vi "_Validate Parameter.vi"(6 "Parameter":T1 {"Expt"."Mass Range"."Resolution Type" items=["High/High", "Medium/Medium", "Low/Low", "High/Medium", "High/Low", "Medium/High", "Medium/Low", "Low/High", "Low/Medium"]}, 9 "error in (no error)":errorcluster) -> (0 "Ch ID":i32[](array[numeric]), 1 "General Param":i32[](array[numeric]), 2 "RunMode":i32, 3 "error out":errorcluster, 4 "Low Values":i32[](array[numeric]), 5 "High Values (DAC)":i32[](array[numeric]))   [LabVIEW 2012]
uses:
  Type/_RT Parameter.ctl
  Type/_RT Active Ch.ctl
  Type/_RT Expt.ctl
  Type/_Run Mode.ctl
  Type/_RT Mass Range.ctl
  Type/_RT Res Type.ctl
  _RT Global.vi
panel:
  # "General Parameters:\n===============\nRun Mode\n# of Ch's\nHigh Level Time (uS) / Q1 Pol\nLow Level Time (uS) / Q2 Pol"
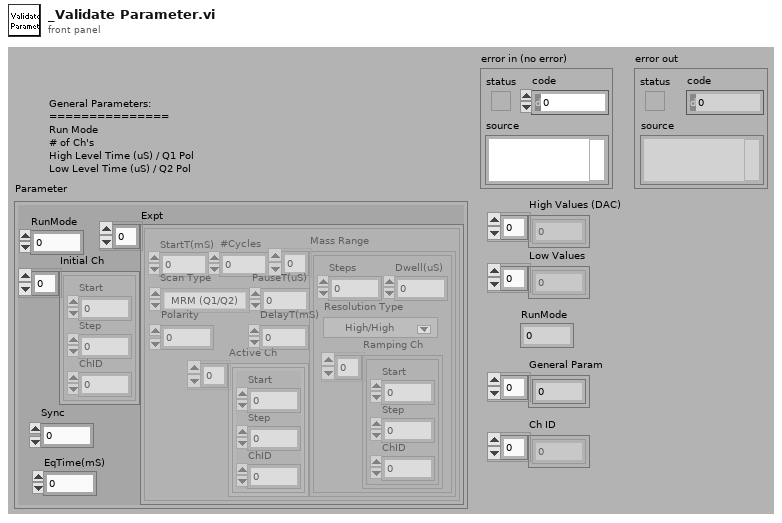
[diagram p1: front panel]
types:
  T1 = typedef "_RT Parameter.ctl" = cluster{"RunMode":i32, "Initial Ch":T2[], "Sync":u8, "Expt":T3[], "EqTime(mS)":i32}
  T2 = typedef "_RT Active Ch.ctl" = cluster{"Start":i32, "Step":i32, "ChID":i32}
  T3 = typedef "_RT Expt.ctl" = cluster{"StartT(mS)":i32, "#Cycles":i32, "Scan Type":T4, "PauseT(uS)":i32, "Polarity":u8, "DelayT(mS)":i32, "Active Ch":T2[], "Mass Range":T5[]}
  T4 = typedef "_Run Mode.ctl" = enum16{"MRM (Q1/Q2)", "Q1 Scan", "Q1 SRM", "Q2 Scan", "Q2 SRM", "Product Scan", "Precursor Scan", "Neutral Loss", "Neutral Gain"}
  T5 = typedef "_RT Mass Range.ctl" = cluster{"Steps":i32, "Dwell(uS)":i32, "Resolution Type":T6, "Ramping Ch":T2[]}
  T6 = typedef "_RT Res Type.ctl" = u16
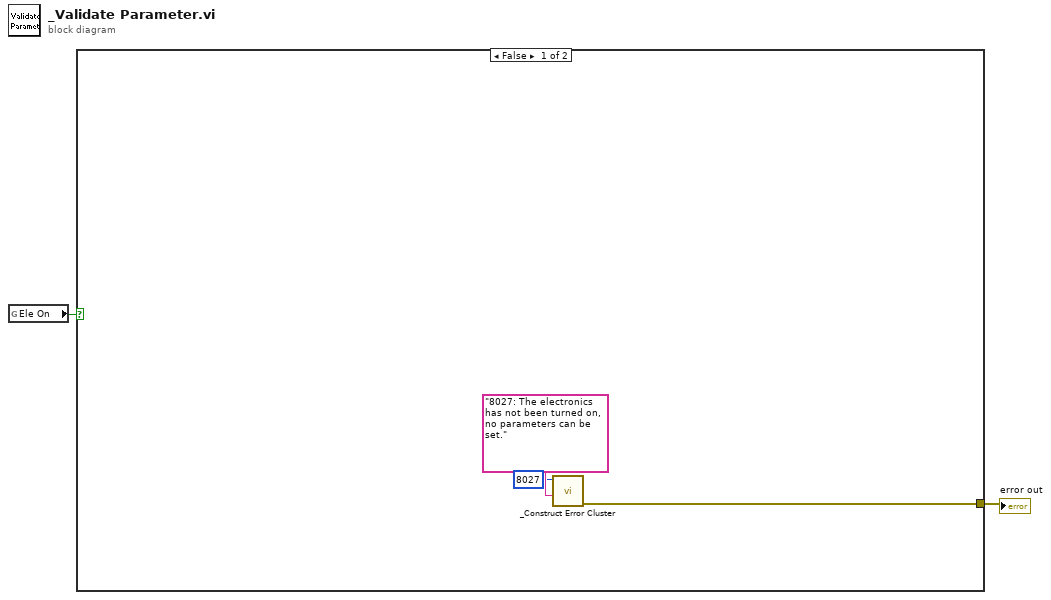
[diagram p0: block diagram]
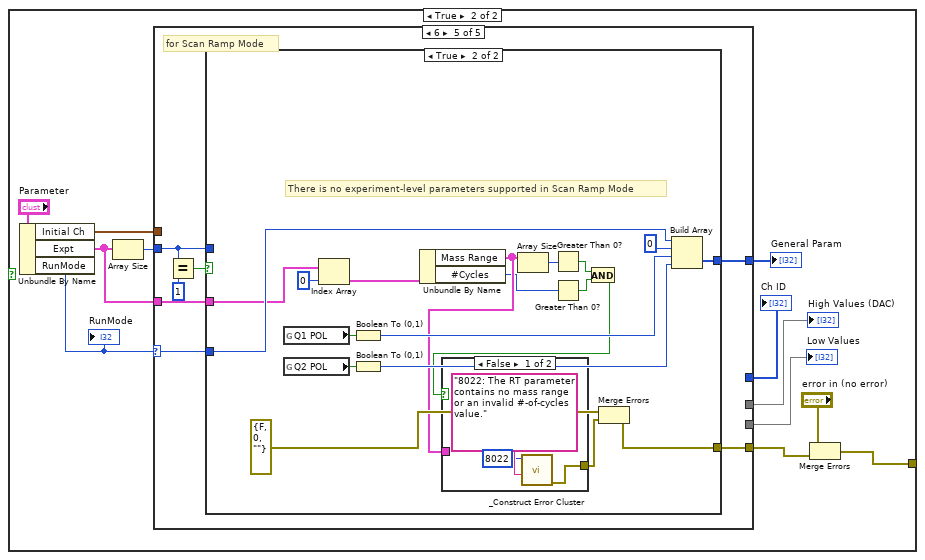
[diagram p2: hidden frame]
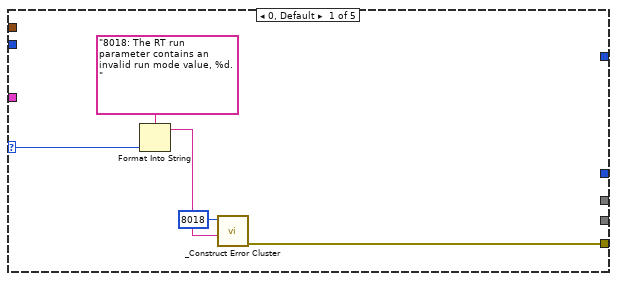
[diagram p3: hidden frame]
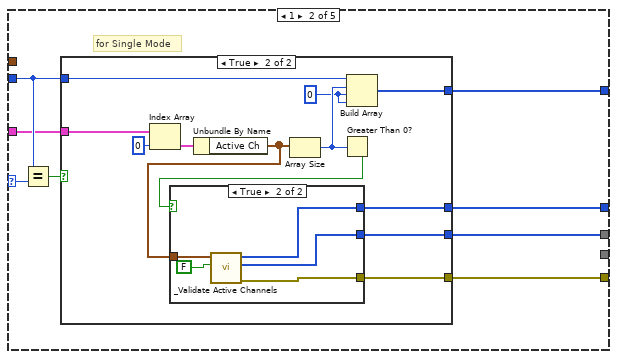
[diagram p4: hidden frame]
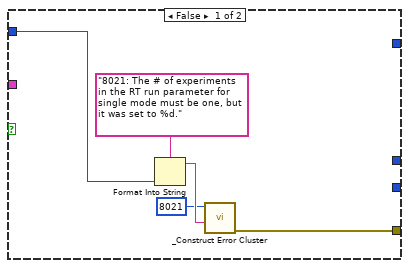
[diagram p5: hidden frame]
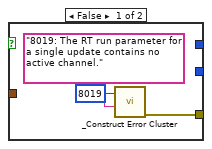
[diagram p6: hidden frame]
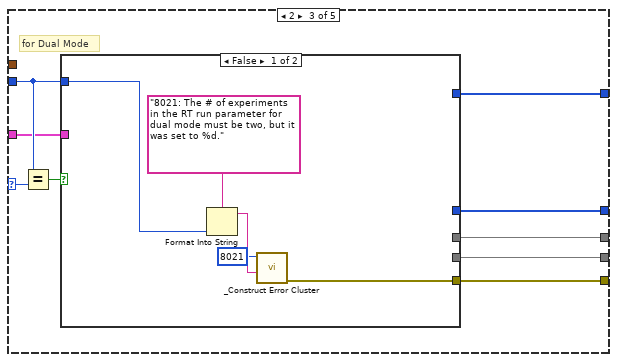
[diagram p7: hidden frame]
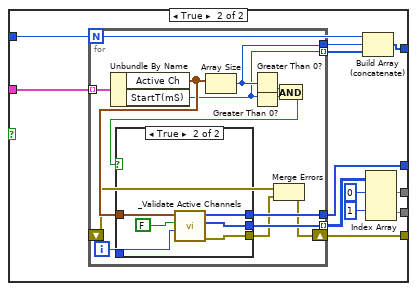
[diagram p8: hidden frame]
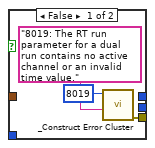
[diagram p9: hidden frame]
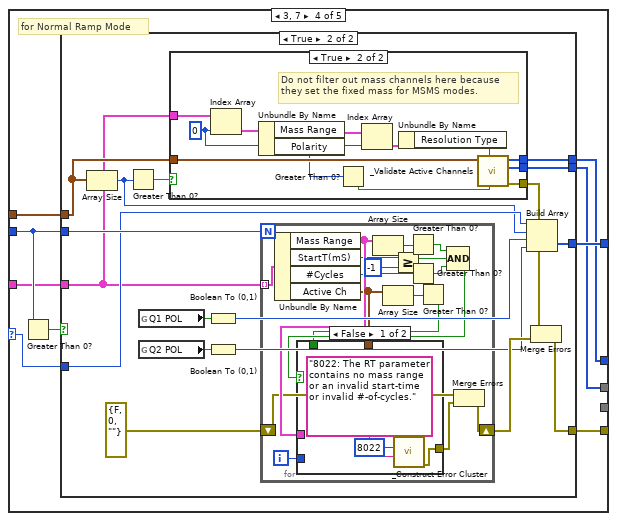
[diagram p10: hidden frame]
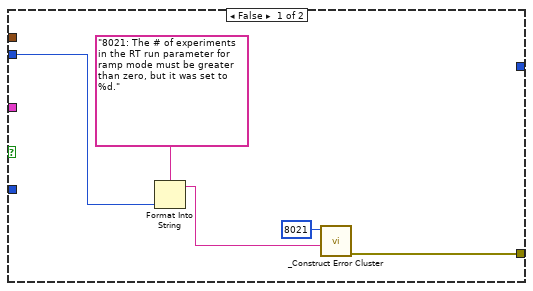
[diagram p11: hidden frame]
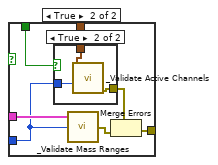
[diagram p13: hidden frame]
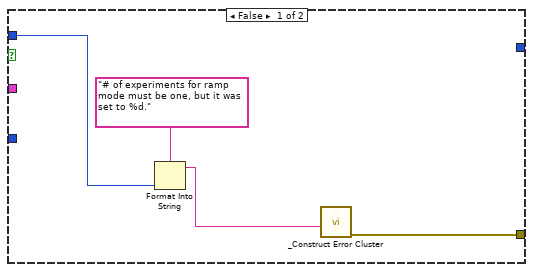
[diagram p15: hidden frame]
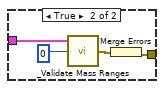
[diagram p16: hidden frame]
diagram:
  n1 = global read "_RT Global.vi" "Ele On"() -> (w1:bool)
  n2 = case shown="False" w1 {
    tunnel: [w3 w13] -> w2
    frame False {
      n3 = call "_Construct Error Cluster.vi"("reason"="8027: The electronics has not been turned on, no parameters can be set.", "errorCode"=8027) -> ("error out"=w3:errorcluster)  [unwired: 2 in, 3 out]
    }
    frame True {
      n4 = Unbundle By Name("Parameter") -> ("Initial Ch"=w6:T2[], "Expt"=w17:T3[], "RunMode"=w7:i32)
      "RunMode" <- w7
      n5 = Array Size(array=w17) -> (size(s)=w16:i32)
      n6 = case shown="6" w7 {
        selector: w7 -> [w21 w28 w62 w104 w179]
        tunnel: [w20 w30 w64 w112 w183] -> w15
        tunnel: w17 -> [_ w26 w60 w109 w181]
        tunnel: w16 -> [_ w27 w61 w110 w178]
        tunnel: [_ w25 w58 w106 _] -> w12
        tunnel: [_ w24 w57 w105 _] -> w11
        tunnel: [_ w23 w59 w108 w180] -> w10
        tunnel: [_ _ w56 _ _] -> w9
        tunnel: w6 -> [_ _ _ w107 _]
        frame 0, Default {
          n7 = Format Into String(format string="8018: The RT run parameter contains an invalid run mode value, %d.", w21) -> (resulting string=w19:string)  [unwired: 2 in, 1 out]
          n8 = call "_Construct Error Cluster.vi"("reason"=w19, "errorCode"=8018) -> ("error out"=w20:errorcluster)  [unwired: 2 in, 3 out]
        }
        frame 1 {
          # "for Single Mode"
          n9 = Equal?(x=w27, y=w28) -> (x = y?=w29:bool)
          n10 = case shown="True" w29 {
            tunnel: [w35 w43] -> w30
            tunnel: w27 -> [w33 w39]
            tunnel: w26 -> [_ w47]
            tunnel: [_ w41] -> w25
            tunnel: [_ w40] -> w24
            tunnel: [_ w36] -> w23
            frame False {
              n11 = Format Into String(format string="8021: The # of experiments in the RT run parameter for single mode must be one, but it was set to %d.", w33) -> (resulting string=w32:string)  [unwired: 2 in, 1 out]
              n12 = call "_Construct Error Cluster.vi"("reason"=w32, "errorCode"=8021) -> ("error out"=w35:errorcluster)  [unwired: 2 in, 3 out]
            }
            frame True {
              w37 = 0 ("element")
              n13 = Index Array(array=w47, index=0) -> (element=w45:T3)
              n14 = Unbundle By Name(w45) -> ("Active Ch"=w42:T2[])
              n15 = Array Size(array=w42) -> (size(s)=w38:i32)
              n16 = Greater Than 0?(x=w38) -> (x > 0?=w44:bool)
              n17 = case shown="True" w44 {
                tunnel: [w49 w55] -> w43
                tunnel: w42 -> [_ w54]
                tunnel: [_ w53] -> w41
                tunnel: [_ w52] -> w40
                frame False {
                  n18 = call "_Construct Error Cluster.vi"("reason"="8019: The RT run parameter for a single update contains no active channel.", "errorCode"=8019) -> ("error out"=w49:errorcluster)  [unwired: 2 in, 3 out]
                }
                frame True {
                  n19 = call "_Validate Active Channels.vi"("User Res Table (T)"=FALSE, "Active Ch"=w54) -> ("error out"=w55:errorcluster, "DAC Values"=w52:i32[], "Ch ID"=w53:i32[])  [unwired: 4 in, 1 out]
                }
              }
              n20 = Build Array(w39, w38, w37, w37) -> (w36:i32[])
            }
          }
        }
        frame 2 {
          # "for Dual Mode"
          n21 = Equal?(x=w61, y=w62) -> (x = y?=w63:bool)
          n22 = case shown="False" w63 {
            tunnel: [w69 w81] -> w64
            tunnel: w61 -> [w67 w78]
            tunnel: w60 -> [_ w80]
            tunnel: [_ w79] -> w59
            tunnel: [_ w75] -> w58
            tunnel: [_ w71] -> w57
            tunnel: [_ w70] -> w56
            frame False {
              n23 = Format Into String(format string="8021: The # of experiments in the RT run parameter for dual mode must be two, but it was set to %d.", w67) -> (resulting string=w66:string)  [unwired: 2 in, 1 out]
              n24 = call "_Construct Error Cluster.vi"("reason"=w66, "errorCode"=8021) -> ("error out"=w69:errorcluster)  [unwired: 2 in, 3 out]
            }
            frame True {
              n25 = for {
                N: w78 -> [_]
                tunnel: w80 -> [w93] mode=indexing
                tunnel: [w89] -> w77
                tunnel: [w88] -> w76 mode=indexing
                tunnel: [w87] -> w75
                tunnel: [w86] -> w74 mode=indexing
                shift-right: [w84] -> w81
                shift-left: _ -> [w83]
                i -> [w82]
                n26 = Unbundle By Name(w93) -> ("Active Ch"=w94:T2[], "StartT(mS)"=w88:i32)
                n27 = Array Size(array=w94) -> (size(s)=w89:i32)
                n28 = Greater Than 0?(x=w89) -> (x > 0?=w91:bool)
                n29 = Greater Than 0?(x=w88) -> (x > 0?=w92:bool)
                n30 = And(x=w91, y=w92) -> (x .and. y?=w90:bool)
                n31 = case shown="True" w90 {
                  tunnel: [w96 w103] -> w85
                  tunnel: w94 -> [_ w102]
                  tunnel: [_ w101] -> w87
                  tunnel: [_ w100] -> w86
                  tunnel: w82 -> [_ w98]
                  frame False {
                    n32 = call "_Construct Error Cluster.vi"("reason"="8019: The RT run parameter for a dual run contains no active channel or an invalid time value.", "errorCode"=8019) -> ("error out"=w96:errorcluster)  [unwired: 2 in, 3 out]
                  }
                  frame True {
                    n33 = call "_Validate Active Channels.vi"("Expt#"=w98, "User Res Table (T)"=FALSE, "Active Ch"=w102) -> ("error out"=w103:errorcluster, "DAC Values"=w100:i32[], "Ch ID"=w101:i32[])  [unwired: 3 in, 1 out]
                  }
                }
                n34 = Merge Errors(w83, w85) -> (w84:errorcluster)
              }
              n35 = Build Array (concatenate)(w78, w77, w76) -> (w79:i32[])
              n36 = Index Array(array=w74, index (row) #1=0 ("index (row)"), index (row) #2=1 ("index (row)")) -> (element #1=w71:i32[], element #2=w70:i32[])  [unwired: 2 in]
            }
          }
        }
        frame 3, 7 {
          # "for Normal Ramp Mode"
          n37 = Greater Than 0?(x=w110) -> (x > 0?=w111:bool)
          n38 = case shown="True" w111 {
            tunnel: [w117 w128] -> w112
            tunnel: w110 -> [w115 w134]
            tunnel: w109 -> [_ w122]
            tunnel: [_ w133] -> w108
            tunnel: w107 -> [_ w131]
            tunnel: [_ w127] -> w106
            tunnel: [_ w126] -> w105
            tunnel: w104 -> [_ w124]
            frame False {
              n39 = Format Into String(format string="8021: The # of experiments in the RT run parameter for ramp mode must be greater than zero, but it was set to %d.", w115) -> (resulting string=w114:string)  [unwired: 2 in, 1 out]
              n40 = call "_Construct Error Cluster.vi"("reason"=w114, "errorCode"=8021) -> ("error out"=w117:errorcluster)  [unwired: 2 in, 3 out]
            }
            frame True {
              n41 = Array Size(array=w131) -> (size(s)=w123:i32)
              n42 = Greater Than 0?(x=w123) -> (x > 0?=w132:bool)
              n43 = global read "_RT Global.vi" "Q1 POL"() -> (w120:bool)
              n44 = global read "_RT Global.vi" "Q2 POL"() -> (w121:bool)
              n45 = case shown="True" w132 {
                tunnel: [_ w146] -> w130
                tunnel: w131 -> [_ w143]
                tunnel: [_ w145] -> w127
                tunnel: [_ w144] -> w126
                tunnel: w122 -> [_ w142]
                frame False {
                }
                frame True {
                  w137 = 0 ("index")
                  # "Do not filter out mass channels here because\nthey set the fixed mass for MSMS modes."
                  n46 = Index Array(array=w142, index=w137) -> (element=w141:T3)
                  n47 = Unbundle By Name(w141) -> ("Mass Range"=w140:T5[], "Polarity"=w136:u8)
                  n48 = Greater Than 0?(x=w136) -> (x > 0?=w135:bool)
                  n49 = Index Array(array=w140, index=w137) -> (element=w139:T5)
                  n50 = Unbundle By Name(w139) -> ("Resolution Type"=w138:T6)
                  n51 = call "_Validate Active Channels.vi"("Negative (F)"=w135, "Resolution Type"=w138, "Active Ch"=w143) -> ("error out"=w146:errorcluster, "DAC Values"=w144:i32[], "Ch ID"=w145:i32[])  [unwired: 3 in, 1 out]
                }
              }
              n52 = Boolean To (0,1)(Boolean=w120) -> (0, 1=w119:i16)
              n53 = Boolean To (0,1)(Boolean=w121) -> (0, 1=w118:i16)
              n54 = for {
                N: w134 -> [_]
                tunnel: w122 -> [w161] mode=indexing
                shift-right: [w152] -> w129
                shift-left: errorcluster {"status"=FALSE, "code"=0, "source"=""} ("error out") -> [w151]
                i -> [w150]
                n55 = Unbundle By Name(w161) -> ("Mass Range"=w162:T5[], "StartT(mS)"=w148:i32, "#Cycles"=w158:i32, "Active Ch"=w154:T2[])
                n56 = Array Size(array=w162) -> (size(s)=w163:i32)
                n57 = Array Size(array=w154) -> (size(s)=w156:i32)
                n58 = Greater Or Equal?(x=w148, y=-1) -> (x >= y?=w149:bool)
                n59 = Greater Than 0?(x=w163) -> (x > 0?=w160:bool)
                n60 = Greater Than 0?(x=w158) -> (x > 0?=w157:bool)
                n61 = Greater Than 0?(x=w156) -> (x > 0?=w155:bool)
                n62 = Compound Arithmetic op=AND(w160, w149, w157) -> (w159:bool)
                n63 = case shown="False" w159 {
                  tunnel: [w165 w170] -> w153
                  tunnel: w162 -> [_ w171]
                  tunnel: w155 -> [_ w173]
                  tunnel: w154 -> [_ w172]
                  tunnel: w150 -> [_ w167]
                  frame False {
                    n64 = call "_Construct Error Cluster.vi"("reason"="8022: The RT parameter contains no mass range or an invalid start-time or invalid #-of-cycles.", "errorCode"=8022) -> ("error out"=w165:errorcluster)  [unwired: 2 in, 3 out]
                  }
                  frame True {
                    n65 = case shown="True" w173 {
                      tunnel: w172 -> [_ w176]
                      tunnel: [_ w175] -> w169
                      tunnel: w167 -> [_ w174]
                      frame False {
                      }
                      frame True {
                        n66 = call "_Validate Active Channels.vi"("Expt#"=w174, "Active Ch"=w176) -> ("error out"=w175:errorcluster)  [unwired: 4 in, 3 out]
                      }
                    }
                    n67 = call "_Validate Mass Ranges.vi"("Expt#"=w167, "Mass Range"=w171) -> ("error out"=w168:errorcluster)  [unwired: 1 in]
                    n68 = Merge Errors(w169, w168) -> (w170:errorcluster)
                  }
                }
                n69 = Merge Errors(w151, w153) -> (w152:errorcluster)
              }
              n70 = Build Array(w124, w123, w119, w118) -> (w133:i32[])
              n71 = Merge Errors(w130, w129) -> (w128:errorcluster)
            }
          }
        }
        frame 6 {
          # "for Scan Ramp Mode"
          n72 = Equal?(x=w178, y=1) -> (x = y?=w182:bool)
          n73 = case shown="True" w182 {
            tunnel: [w187 w198] -> w183
            tunnel: w178 -> [w185 _]
            tunnel: w181 -> [_ w190]
            tunnel: [_ w206] -> w180
            tunnel: w179 -> [_ w204]
            frame False {
              n74 = Format Into String(format string="# of experiments for ramp mode must be one, but it was set to %d.", w185) -> (resulting string=w184:string)  [unwired: 2 in, 1 out]
              n75 = call "_Construct Error Cluster.vi"("reason"=w184) -> ("error out"=w187:errorcluster)  [unwired: 3 in, 3 out]
            }
            frame True {
              # "There is no experiment-level parameters supported in Scan Ramp Mode"
              n76 = global read "_RT Global.vi" "Q1 POL"() -> (w202:bool)
              n77 = global read "_RT Global.vi" "Q2 POL"() -> (w203:bool)
              n78 = Index Array(array=w190, index=0) -> (element=w188:T3)
              n79 = Boolean To (0,1)(Boolean=w202) -> (0, 1=w201:i16)
              n80 = Boolean To (0,1)(Boolean=w203) -> (0, 1=w200:i16)
              n81 = Unbundle By Name(w188) -> ("Mass Range"=w196:T5[], "#Cycles"=w193:i32)
              n82 = Array Size(array=w196) -> (size(s)=w197:i32)
              n83 = Greater Than 0?(x=w197) -> (x > 0?=w195:bool)
              n84 = Greater Than 0?(x=w193) -> (x > 0?=w192:bool)
              n85 = And(x=w195, y=w192) -> (x .and. y?=w194:bool)
              n86 = case shown="False" w194 {
                tunnel: [w208 w212] -> w191
                tunnel: w196 -> [_ w213]
                frame False {
                  n87 = call "_Construct Error Cluster.vi"("reason"="8022: The RT parameter contains no mass range or an invalid #-of-cycles value.", "errorCode"=8022) -> ("error out"=w208:errorcluster)  [unwired: 2 in, 3 out]
                }
                frame True {
                  n88 = call "_Validate Mass Ranges.vi"("Expt#"=0, "Mass Range"=w213) -> ("error out"=w211:errorcluster)  [unwired: 1 in]
                  n89 = Merge Errors(w211) -> (w212:errorcluster)
                }
              }
              n90 = Merge Errors(errorcluster {"status"=FALSE, "code"=0, "source"=""} ("error out"), w191) -> (w198:errorcluster)
              n91 = Build Array(w204, 0 ("size(s)"), w201, w200) -> (w206:i32[])
            }
          }
        }
      }
      "General Param" <- w10
      "Ch ID" <- w12
      "High Values (DAC)" <- w11
      "Low Values" <- w9
      n92 = Merge Errors("error in (no error)", w15) -> (w13:errorcluster)
    }
  }
  "error out" <- w2
